vi "Draw Button.vi"(6 "Force redraw ?":bool, 7 "Button State":T2, 8 "error in (no error)":errorcluster, 9 "Button Style":T1=enum."Classic", 10 "Button Size":i32, 11 "Button.lvclass":refnum<class "Button.lvclass">) -> (0 "error out":errorcluster, 1 "Picture Out":picture, 2 "Image (no button)":picture, 3 "Button.lvclass Out":refnum<class "Button.lvclass">)   [LabVIEW 2012, in "Button.lvclass"]
doc: "Public method of the button class to draw itself given the button size, style(system, flat, rounded etc) and state (on, off, hover)"
uses:
  Button.lvclass
  Type Defs/Button Status.ctl
  Type Defs/Button Style.ctl
  Button.lvclass/Button.ctl
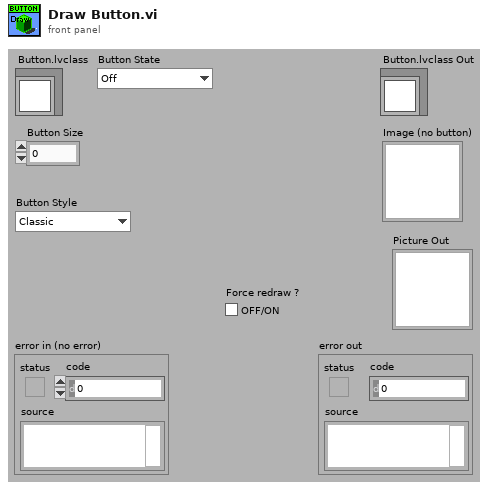
[diagram p1: front panel]
types:
  T1 = typedef "Button.lvclass/Button Style.ctl" = enum16{"System", "Modern", "Classic", "Rounded", "Silver", "Ni Theme", "Metallic"}
  T2 = typedef "Button.lvclass/Button Status.ctl" = enum16{"Off", "Hover", "On", "Disabled"}
  T3 = typedef "imagedata.ctl" = cluster{"image type":i32, "image depth":i32, "image":u8[], "mask":u8[], "colors":u32[], "Rectangle":cluster{"left":i16, "top":i16, "right":i16, "bottom":i16}}
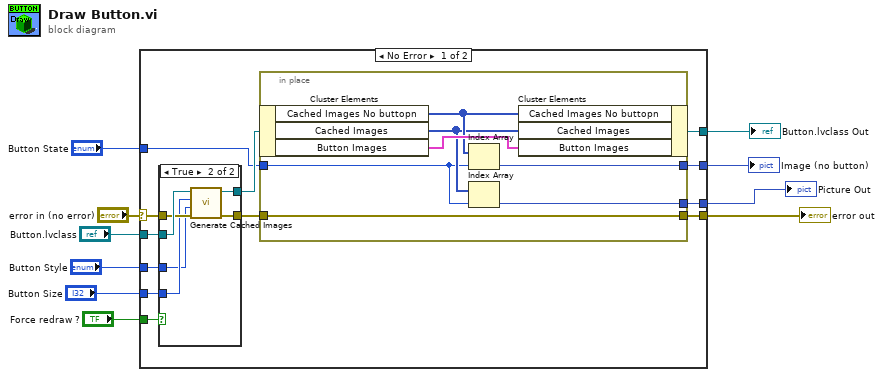
[diagram p0: block diagram]
diagram:
  n1 = case shown="No Error" "error in (no error)" {
    selector: "error in (no error)" -> [w16 w39]
    tunnel: "Button State" -> [w11 _]
    tunnel: [w22 w39] -> w9
    tunnel: "Button.lvclass" -> [w21 w38]
    tunnel: "Button Style" -> [w12 _]
    tunnel: "Button Size" -> [w13 _]
    tunnel: [w20 w38] -> w4
    tunnel: "Force redraw ?" -> [w14 _]
    tunnel: [w19 _] -> w2
    tunnel: [w18 _] -> w1
    frame No Error {
      n2 = case shown="True" w14 {
        tunnel: w21 -> [w24 w30]
        tunnel: [w24 w29] -> w17
        tunnel: w16 -> [w23 w28]
        tunnel: [w23 w27] -> w15
        tunnel: w13 -> [_ w26]
        tunnel: w12 -> [_ w25]
        frame False {
        }
        frame True {
          n3 = call-dynamic "Generate Cached Images.vi"("error in (no error)"=w28, "Button Style"=w25, "Button Size"=w26, "object in"=w30) -> ("error out"=w27:errorcluster, "object out"=w29:refnum<class "Button.lvclass">)  [unwired: 6 in]
        }
      }
      n4 = in-place {
        in-place-border: [w36] -> w22
        in-place-border: w15 -> [w36]
        in-place-border: w11 -> [w32]
        in-place-border: [w34] -> w19
        in-place-border: [w31] -> w18
        n5 = in-place-cluster #1(w17) -> ("Cached Images No buttopn"=w35:picture[], "Cached Images"=w33:picture[], "Button Images"=w37:T3[])
        n6 = Index Array(array=w35, index=w32) -> (element=w34:picture)
        n7 = Index Array(array=w33, index=w32) -> (element=w31:picture)
        n8 = in-place-cluster #1("Cached Images No buttopn"=w35, "Cached Images"=w33, "Button Images"=w37) -> (w20:refnum<class "Button.lvclass">)
      }
    }
    frame Error {
    }
  }
  "Picture Out" <- w1
  "error out" <- w9
  "Image (no button)" <- w2
  "Button.lvclass Out" <- w4
